vi "From Byte Array (LV Timestamp).vi"(1 "byte array in":u8[](array[numeric]) format="%x") -> (0 "element out":timestamp)   [LabVIEW 2013]
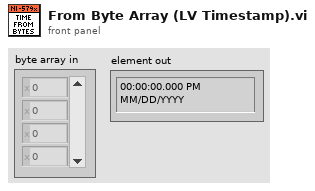
[diagram p1: front panel]
types:
  T1 = enum16{"big-endian, network order", "native, host order", "little-endian"}
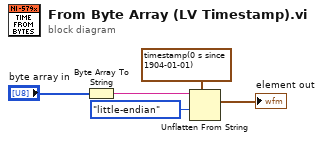
[diagram p0: block diagram]
diagram:
  n1 = Byte Array To String(unsigned byte array="byte array in") -> (string=w5:string)
  n2 = Unflatten From String(type=timestamp(0 s since 1904-01-01), binary string=w5, byte order (0:big-endian, network order)=T1."little-endian") -> (value=→"element out":timestamp)  [unwired: 2 in, 2 out]
